vi "Main v1.5.vi"() -> ()   [LabVIEW 2017]
doc: "v0.85:\n- Counts for rejects and total\n\nv0.5:\n\n- Added Reject to Manual Mode\n- Send reject pallet cluster during manual mode\n- Run continuous manual happens only when no error has occured"
uses:
  Controls/Main Tabs v0.1.ctl
  Controls/Auto.ctl
  RT/Controls/Auto Delays.ctl
  RT/Controls/Auto Times.ctl
  support/Controls/General Para.ctl
  Controls/UI Data.ctl
  support/Controls/Auto Stats.ctl
  Controls/Logging FGV.ctl
  support/Message Queue/Enqueue Message (Single).vi
  GV/Maintenance GV.vi
  <vilib>/Utility/error.llb/Error Cluster From Error Code.vi
  <vilib>/ErrorRing/Error Ring.xnode
  support/Message Queue/Message Queue.lvlib
  support/User Event - Stop/User Event - Stop.lvlib
panel:
  out "path":path
  in  "General Para 2":T1={"Max. Cons."=5.0, "Offset 1"=0.0, "Offset 2"=0.0, "Offset 3"=0.0, "Offset 4"=-0.6, "OutputPause"=500.0, "RejectPause"=500.0} caption="General Para" {"Offset 4" format="%.2f"; "Offset 3" format="%.2f"; "Offset 2" format="%.2f"; "Offset 1" format="%.2f"}
  in  "Auto Para 2":T2={"Agitator Delays"=[250, 600], "TF Delays"=[400, 800, 2, 8000], "Insertion Delays"=[100, 400], "Cutting Delays"=[200, 300, 50], "PF Delays"=[300, 8000], "Measur. Delays"=[200.0, 188.9, 1.0], "Reject Delays"=[500], "BF Delays"=[1000, 1000]}
  out "Shutdown?":bool
  out "Boolean 8":bool
  out "Boolean 7":bool
  out "Boolean 6":bool
  out "Boolean 5":bool
  out "Boolean 4":bool
  out "Boolean 3":bool
  out "Boolean 2":bool
  out "Boolean":bool
  in  "Reject Pallets":T3
  out "Date-Time":string caption="Dip-Tube Assembly Automation (HMI) v1.5"
  out "Main Tab":T4
  in  "All IOs":bool
  in  "Autocycle":T5
  in  "Manual":bool
  in  "Parameters":bool
  in  "Maintenance":bool
  in  "General Para":T1={"Max. Cons."=5.0, "Offset 1"=0.0, "Offset 2"=0.0, "Offset 3"=0.0, "Offset 4"=0.0, "OutputPause"=0.0, "RejectPause"=0.0} {"Offset 4" format="%.2f"; "Offset 3" format="%.2f"; "Offset 2" format="%.2f"; "Offset 1" format="%.2f"}
  in  "BF Para":cluster{"Delay 1":u32, "Delay 2":u32}={"Delay 1"=1000, "Delay 2"=1000}
  in  "Reject Para":cluster{"Delay":u32}={"Delay"=400}
  in  "Meas. Para":T6={"Delay"=500.0, "Mean Length"=188.9, "Tolerance"=1.0}
  in  "PF Para":cluster{"Delay":u32, "Timeout":u32}={"Delay"=1000, "Timeout"=1000}
  in  "Tube Feeder Para":T7={"Delay"=400, "Delay 2"=250, "Max Attempts"=250, "Timeout"=8000}
  in  "Cutting Para":T8={"Delay"=400, "Delay 2"=250, "Delay 3"=250}
  in  "Agitator Para":cluster{"Delay":u32, "Timeout":u32}={"Delay"=400, "Timeout"=250}
  in  "Insertion Para":cluster{"Delay 1":u32, "Delay 2":u32}={"Delay 1"=1000, "Delay 2"=1000}
  in  "Save Para":bool
  in  "Home Para":bool
  out "OEE":dbl format="%#.1f"
  out "QUA":dbl=100.0 min=0.0 max=100.0 step=0.1
  in  "Ideal Time":dbl=2.0 min=0.0 max=100.0 step=0.1
  in  "AVL":dbl=100.0 min=0.0 max=100.0 step=0.1
  out "Rejects 2":u32 caption="Rejects"
  in  "Reset MCount":bool
  in  "Enable BF?":bool
  in  "Enable Agitate?":bool
  in  "Enable Reject?":bool
  in  "Toggle Motor":bool
  in  "Continuous?":bool
  in  "Enable Measure?":bool
  in  "Enable Index?":bool
  in  "Enable PF?":bool
  in  "Manual Para":T2={"Agitator Delays"=[400, 250], "TF Delays"=[700, 800, 2], "Insertion Delays"=[100, 500], "Cutting Delays"=[300, 300, 100], "PF Delays"=[250, 30000], "Measur. Delays"=[500.0, 188.9, 1.0], "Reject Delays"=[500], "BF Delays"=[1000, 1000]}
  in  "Enable Cutting?":bool
  in  "Enable Insertion?":bool
  in  "Run Manual":bool
  in  "Enable TF?":bool
  in  "Home Manual":bool
  out "Status 2":T10
  out "Measurements":T11 {"Height 1" format="%#.2f"; "Height 2" format="%#.2f"; "Height 3" format="%#.2f"; "Height 4" format="%#.2f"}
  out "Output Count":u32 caption="Output\nCount"
  out "PRF":dbl=100.0 min=0.0 max=100.0 step=0.1
  in  "End Cycle":bool
  out "Statuses":string[][](table)
  in  "All IO":bool
  in  "Stats":bool
  in  "Home AC":bool
  out "Status":string
  out "Good":u32 format="%06.0f"
  out "Cycle Time":dbl format="%0.2f"
  out "Rejects":u32 format="%06.0f"
  in  "View Log":bool
  out "Total Count 2":u32 caption="Total Count"
  out "Avg. Time":dbl caption="Avg. Cycle Time (s)" format="%#.3f"
  out "Output Chart":cluster{"Good Parts":u32, "Reject Parts":u32}(graph)
  out "Reject Count":u32
  out "Good Count":u32
  out "Total Time":dbl caption="Effective Cycle Time (s)" format="%#.3f"
  out "Time Chart":T12(graph)
  out "OEE Chart":T13(graph)
  out "Timestamp":string caption="Date & Timestamp"
  out "Latest Measure.":T14 caption="Latest Measurements" {"Length 1 (mm)" format="%#.2f"}
  out "Auto Times":T9
  in  "Back Stats":bool
  out "OEE 2":T13 caption="Latest Measurements" {"AVL" format="%#.1f"; "PRF" format="%#.1f"; "QUA" format="%#.1f"; "OEE" format="%#.1f"}
  out "Measurement Chart":T15(graph)
  in  "Home IOs":bool
  in  "Back IO":bool
  out "IAS 4":dbl format="%#.3f"
  out "IAS 3":dbl format="%#.3f"
  out "IAS 2":dbl format="%#.3f"
  out "IAS 1":dbl format="%#.3f"
  out "DI 1":T16
  out "DI 2":T17
  out "DO 1":T18
  in  "Exit":bool
  in  "Shutdown":bool
  # "HARMONY VISION DIP-TUBE ASSEMBLY AUTOMATION"
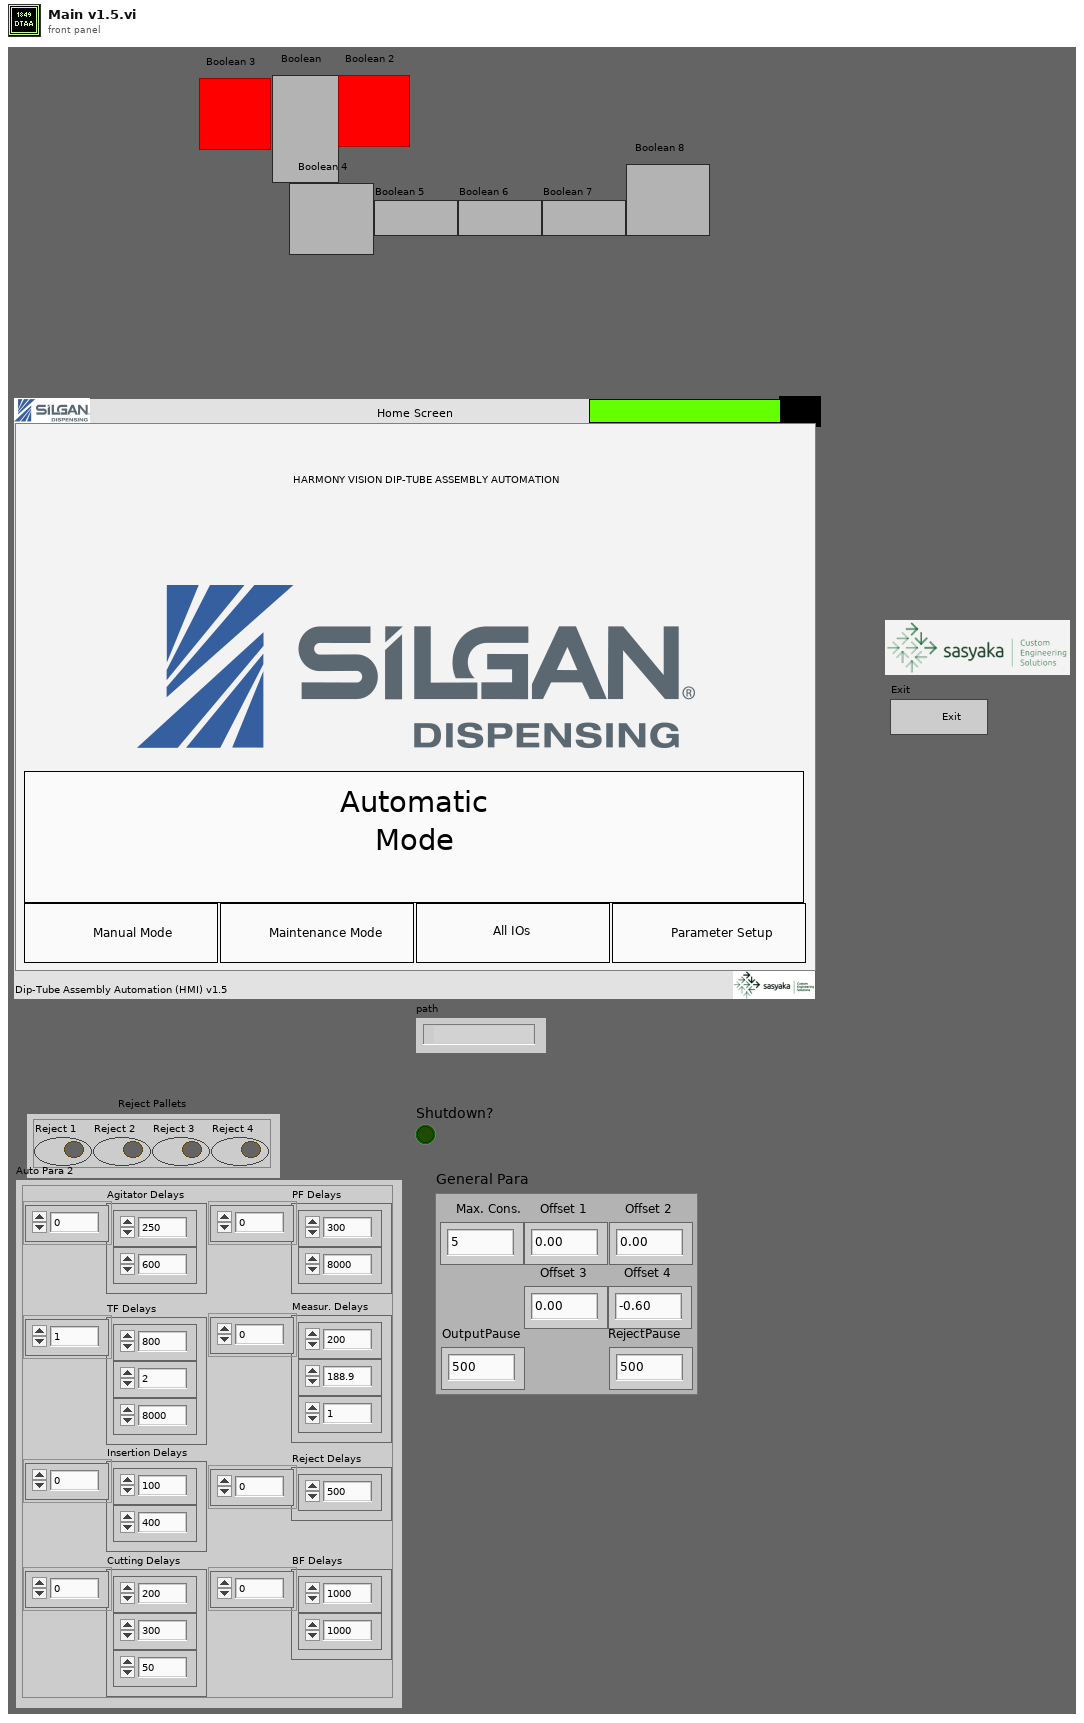
[diagram p1: front panel]
types:
  T1 = typedef "General Para.ctl" = cluster{"Max. Cons.":dbl, "Offset 1":dbl, "Offset 2":dbl, "Offset 3":dbl, "Offset 4":dbl, "OutputPause":dbl, "RejectPause":dbl}
  T2 = typedef "Auto Delays.ctl" = cluster{"Agitator Delays":u32[], "TF Delays":u32[], "Insertion Delays":u32[], "Cutting Delays":u32[], "PF Delays":u32[], "Measur. Delays":dbl[], "Reject Delays":u32[], "BF Delays":u32[]}
  T3 = cluster{"Reject 1":bool, "Reject 2":bool, "Reject 3":bool, "Reject 4":bool}
  T4 = typedef "Main Tabs v0.1.ctl" = enum32{"Home Screen", "Parameter Setup", "Manual Mode", "Autocycle", "Autocycle Statistics", "Autocycle IOs"}
  T5 = typedef "Auto.ctl" = bool
  T6 = cluster{"Delay":dbl, "Mean Length":dbl, "Tolerance":dbl}
  T7 = cluster{"Delay":u32, "Delay 2":u32, "Max Attempts":u32, "Timeout":u32}
  T8 = cluster{"Delay":u32, "Delay 2":u32, "Delay 3":u32}
  T9 = typedef "Auto Times.ctl" = cluster{"Index Time":u32, "TF Time":u32, "Insertion Time":u32, "Cutting Time":u32, "PF Time":u32, "Meas. Time":u32, "Reject Time":u32}
  T10 = cluster{"Auto Times":T9, "error out":errorcluster}
  T11 = cluster{"Height 1":dbl, "Height 2":dbl, "Height 3":dbl, "Height 4":dbl}
  T12 = cluster{"Index":dbl, "TF":dbl, "Insert":dbl, "Cutting":dbl, "PF":dbl, "Measure.":dbl, "Reject":dbl}
  T13 = cluster{"AVL":dbl, "PRF":dbl, "QUA":dbl, "OEE":dbl}
  T14 = cluster{"Length 1 (mm)":dbl, "Pallet 2 (mm)":dbl, "Pallet 3 (mm)":dbl, "Pallet 4 (mm)":dbl}
  T15 = cluster{"1":dbl, "2":dbl, "3":dbl, "4":dbl, "4":dbl, "4":dbl}
  T16 = cluster{"Machine_ON":bool, "E_stop ":bool, "SW_Pressure":bool, "SW_Start ":bool, "SW_Reset":bool, "SW_Stop":bool, "SW_Door":bool, "RS_Index_Rotary_CW":bool, "RS_Index_Rotary_CCW":bool, "RS_Index_Stopper _Rear":bool, "RS_Index_Output_Separator_Rear":bool, "PES_Index_Pallet_Sensor":bool, "PES_Index_Output_Part Sensor":bool, "ICS_BF_Low_Level_1":bool, "ICS_BF_Low_Level_2":bool, "ICS_BF_Pump_CNVR_Full_1":bool, "ICS_BF_Pump_CNVR_Full_2":bool, "ICS_BF_Pump_CNVR_Full_3":bool, "ICS_BF_Pump_CNVR_Full_4":bool, "PES_PC_Pump Presence_1":bool, "PES_PC_Pump Presence_2":bool, "PES_PC_Pump Presence_3":bool, "PES_PC_Pump Presence_4":bool, "RS_PC_Gating_Front":bool, "PES_Pump_Interference":bool, "PES_TF_Low_Level":bool, "PES_Tube Presence_1":bool, "PES_Tube Presence_2":bool, "PES_Tube Presence_3":bool, "PES_Tube Presence_4":bool, "DI1.30":bool, "DI1.31":bool}
  T17 = cluster{"RS_Agitatator_1_Rear ":bool, "RS_Agitatator_2_Rear ":bool, "RS_TF_Gating CYL_Rear":bool, "RS_Insertion_1_Rear":bool, "RS_Insertion_1_Front":bool, "RS_Insertion _2_Rear":bool, "RS_Insertion _2_Front":bool, "RS_Insertion _3_Rear":bool, "RS_Insertion _3_Front":bool, "RS_Insertion _4_Rear":bool, "RS_Insertion _4_Front":bool, "RS_Insertion_Clamp_Rear":bool, "RS_Cutting_Rear":bool, "RS_Cutting_Clamp _Rear":bool, "RS_Measurement_1_Rear":bool, "RS_Measurement_2_Rear":bool, "RS_Measurement_3_Rear":bool, "RS_Measurement_4_Rear":bool, "DI2.18":bool, "RS_Rejection_1_Rear":bool, "RS_Rejection_2_Rear":bool, "RS_Rejection_3_Rear":bool, "RS_Rejection_4_Rear":bool, "DI2.23":bool, "DI2.24":bool, "DI2.25":bool, "DI2.26":bool, "DI2.27":bool, "DI2.28":bool, "DI2.29":bool, "DI2.30":bool, "DI2.31":bool}
  T18 = cluster{"TL_Red":bool, "TL_Orange":bool, "TL_Green":bool, "TL_Buzzer":bool, "SOL_Index_Rotary_CW":bool, "SOL_Index_Rotary_CCW":bool, "SOL_Index_Stopper_Rear":bool, "SOL_OutputSeparator_Rear":bool, "Bowl  Feeder_ ON 1":bool, "Pump_CNVR_Motor _ON":bool, "SOL_PC_Gating_CYL_Rear":bool, "SOL_Tube_Feed_Agitatator":bool, "SOL_Tube_Feed_Gating_CYL":bool, "SOL_Insertion _CYL":bool, "SOL_Insertion_Clamp_CYL":bool, "SOL_Cutting_CYL":bool, "SOL_Cutting_Clamp_CYL":bool, "SOL_Insertion_Air_Nozzle":bool, "SOL_Measurement_CYL":bool, "DO1.19":bool, "SOL_Rejection CYL_1":bool, "SOL_Rejection CYL_2":bool, "SOL_Rejection CYL_3":bool, "SOL_Rejection CYL_4":bool, "Bowl  Feeder_ ON 2":bool, "SOL_BF_BlowerON":bool, "SOL_BF1_Track1":bool, "SOL_BF1_Track2":bool, "SOL_BF2_Track1":bool, "SOL_BF2_Track2":bool, "DO1.30":bool, "DO1.31":bool}
  T19 = typedef "UI Data.ctl" = cluster{"Main Tab":refnum<vi>}
  T20 = typedef "Message Queue.lvlib/All Message Queues.ctl" = cluster{"UI":refnum<queue>}
  T21 = enum8{"Enabled", "Disabled", "Disabled and Grayed Out"}
  T22 = cluster{"Array":string[][], "Machine Status":string}
  T23 = typedef "Logging FGV.ctl" = enum16{"Start Shift", "Log Index", "Read Shift", "Close Shift"}
  T24 = typedef "Auto Stats.ctl" = cluster{"Time-Stamp":timestamp, "Auto Times":T9, "Measurements":cluster{"1":dbl, "2":dbl, "3":dbl, "4":dbl}, "Outputs":cluster{"Good Parts":u32, "Reject Parts":u32}, "Cycle Time":dbl, "Remarks":string}
  T25 = cluster{"Auto Times":T9, "Results":cluster{"Measurements":cluster{"1":dbl, "2":dbl, "3":dbl, "4":dbl}, "Reject Pallets":cluster{"Reject 1":bool, "Reject 2":bool, "Reject 3":bool, "Reject 4":bool}}, "OutputCount":u32, "error out":errorcluster}
  T26 = enum8{"Information", "Error", "Successful", "Tips"}
  T27 = cluster{"Agitator Delays[0]":u32, "Agitator Delays[1]":u32}
  T28 = cluster{"TF Delays[0]":u32, "TF Delays[1]":u32, "TF Delays[2]":u32, "TF Delays[3]":u32}
  T29 = cluster{"Insertion Delays[0]":u32, "Insertion Delays[1]":u32}
  T30 = cluster{"Cutting Delays[0]":u32, "Cutting Delays[1]":u32, "Cutting Delays[2]":u32}
  T31 = cluster{"Measur. Delays[0]":dbl, "Measur. Delays[1]":dbl, "Measur. Delays[2]":dbl}
  T32 = typedef "All Inputs.ctl" = cluster{"DI 1":cluster{"Machine_ON":bool, "E_stop ":bool, "SW_Pressure":bool, "SW_Start ":bool, "SW_Reset":bool, "SW_Stop":bool, "SW_Door":bool, "RS_Index_Rotary_CW":bool, "RS_Index_Rotary_CCW":bool, "RS_Index_Stopper _Rear":bool, "RS_Cutting_DNClamp _Rear":bool, "PES_Index_Pallet_Sensor":bool, "PES_Index_Output_Part Sensor":bool, "ICS_BF_Low_Level_1":bool, "ICS_BF_Low_Level_2":bool, "ICS_BF_Pump_CNVR_Full_1":bool, "ICS_BF_Pump_CNVR_Full_2":bool, "ICS_BF_Pump_CNVR_Full_3":bool, "ICS_BF_Pump_CNVR_Full_4":bool, "PES_PC_Pump Presence_1":bool, "PES_PC_Pump Presence_2":bool, "PES_PC_Pump Presence_3":bool, "PES_PC_Pump Presence_4":bool, "RS_PC_Gating_Front":bool, "PES_Pump_Interference":bool, "PES_TF_Low_Level":bool, "PES_Tube Presence_1":bool, "PES_Tube Presence_2":bool, "PES_Tube Presence_3":bool, "PES_Tube Presence_4":bool, "DI1.30":bool, "DI1.31":bool}, "DI 2":cluster{"RS_Agitatator_1_Rear ":bool, "RS_Agitatator_2_Rear ":bool, "RS_TF_Gating CYL_Rear":bool, "RS_Insertion_1_Rear":bool, "RS_Insertion_1_Front":bool, "RS_Insertion _2_Rear":bool, "RS_Insertion _2_Front":bool, "RS_Insertion _3_Rear":bool, "RS_Insertion _3_Front":bool, "RS_Insertion _4_Rear":bool, "RS_Insertion _4_Front":bool, "RS_Insertion_Clamp_Rear":bool, "RS_Cutting_Rear":bool, "RS_Cutting_UPClamp _Rear":bool, "RS_Measurement_1_Rear":bool, "RS_Measurement_2_Rear":bool, "RS_Measurement_3_Rear":bool, "RS_Measurement_4_Rear":bool, "RS_Measure_Clamp_Rear":bool, "RS_Rejection_1_Rear":bool, "RS_Rejection_2_Rear":bool, "RS_Rejection_3_Rear":bool, "RS_Rejection_4_Rear":bool, "DI2.23":bool, "DI2.24":bool, "DI2.25":bool, "DI2.26":bool, "DI2.27":bool, "DI2.28":bool, "DI2.29":bool, "DI2.30":bool, "DI2.31":bool}, "IAS 1":dbl, "IAS 2":dbl, "IAS 3":dbl, "IAS 4":dbl, "DO 1":cluster{"TL_Red":bool, "TL_Orange":bool, "TL_Green":bool, "TL_Buzzer":bool, "SOL_Index_Rotary_CW":bool, "SOL_Index_CNVR_Rotary_CCW":bool, "SOL_Index_CNVR_Stopper_Rear":bool, "SOL_Index_CNVR_Output _Separator _Rear":bool, "Bowl  Feeder_ ON 1":bool, "Pump_CNVR_Motor _ON":bool, "SOL_PC_Gating_CYL_Rear":bool, "SOL_Tube_Feed_Agitatator":bool, "SOL_Tube_Feed_Gating_CYL":bool, "SOL_Insertion _CYL":bool, "SOL_Insertion_Clamp_CYL":bool, "SOL_Cutting_CYL":bool, "SOL_Cutting_Clamp_CYL":bool, "SOL_Insertion_Air_Nozzle":bool, "SOL_Measurement_CYL":bool, "DO1.19":bool, "SOL_Rejection CYL_1":bool, "SOL_Rejection CYL_2":bool, "SOL_Rejection CYL_3":bool, "SOL_Rejection CYL_4":bool, "Bowl  Feeder_ ON 2":bool, "SOL_BF_BlowerON":bool, "SOL_BF1_Track1":bool, "SOL_BF1_Track2":bool, "SOL_BF2_Track1":bool, "SOL_BF2_Track2":bool, "DO1.30":bool, "DO1.31":bool}}
  T33 = cluster{"Machine_ON":bool, "E_stop ":bool, "SW_Pressure":bool, "SW_Start ":bool, "SW_Reset":bool, "SW_Stop":bool, "SW_Door":bool, "RS_Index_Rotary_CW":bool, "RS_Index_Rotary_CCW":bool, "RS_Index_Stopper _Rear":bool, "RS_Cutting_DNClamp _Rear":bool, "PES_Index_Pallet_Sensor":bool, "PES_Index_Output_Part Sensor":bool, "ICS_BF_Low_Level_1":bool, "ICS_BF_Low_Level_2":bool, "ICS_BF_Pump_CNVR_Full_1":bool, "ICS_BF_Pump_CNVR_Full_2":bool, "ICS_BF_Pump_CNVR_Full_3":bool, "ICS_BF_Pump_CNVR_Full_4":bool, "PES_PC_Pump Presence_1":bool, "PES_PC_Pump Presence_2":bool, "PES_PC_Pump Presence_3":bool, "PES_PC_Pump Presence_4":bool, "RS_PC_Gating_Front":bool, "PES_Pump_Interference":bool, "PES_TF_Low_Level":bool, "PES_Tube Presence_1":bool, "PES_Tube Presence_2":bool, "PES_Tube Presence_3":bool, "PES_Tube Presence_4":bool, "DI1.30":bool, "DI1.31":bool}
  T34 = cluster{"RS_Agitatator_1_Rear ":bool, "RS_Agitatator_2_Rear ":bool, "RS_TF_Gating CYL_Rear":bool, "RS_Insertion_1_Rear":bool, "RS_Insertion_1_Front":bool, "RS_Insertion _2_Rear":bool, "RS_Insertion _2_Front":bool, "RS_Insertion _3_Rear":bool, "RS_Insertion _3_Front":bool, "RS_Insertion _4_Rear":bool, "RS_Insertion _4_Front":bool, "RS_Insertion_Clamp_Rear":bool, "RS_Cutting_Rear":bool, "RS_Cutting_UPClamp _Rear":bool, "RS_Measurement_1_Rear":bool, "RS_Measurement_2_Rear":bool, "RS_Measurement_3_Rear":bool, "RS_Measurement_4_Rear":bool, "RS_Measure_Clamp_Rear":bool, "RS_Rejection_1_Rear":bool, "RS_Rejection_2_Rear":bool, "RS_Rejection_3_Rear":bool, "RS_Rejection_4_Rear":bool, "DI2.23":bool, "DI2.24":bool, "DI2.25":bool, "DI2.26":bool, "DI2.27":bool, "DI2.28":bool, "DI2.29":bool, "DI2.30":bool, "DI2.31":bool}
  T35 = cluster{"TL_Red":bool, "TL_Orange":bool, "TL_Green":bool, "TL_Buzzer":bool, "SOL_Index_Rotary_CW":bool, "SOL_Index_CNVR_Rotary_CCW":bool, "SOL_Index_CNVR_Stopper_Rear":bool, "SOL_Index_CNVR_Output _Separator _Rear":bool, "Bowl  Feeder_ ON 1":bool, "Pump_CNVR_Motor _ON":bool, "SOL_PC_Gating_CYL_Rear":bool, "SOL_Tube_Feed_Agitatator":bool, "SOL_Tube_Feed_Gating_CYL":bool, "SOL_Insertion _CYL":bool, "SOL_Insertion_Clamp_CYL":bool, "SOL_Cutting_CYL":bool, "SOL_Cutting_Clamp_CYL":bool, "SOL_Insertion_Air_Nozzle":bool, "SOL_Measurement_CYL":bool, "DO1.19":bool, "SOL_Rejection CYL_1":bool, "SOL_Rejection CYL_2":bool, "SOL_Rejection CYL_3":bool, "SOL_Rejection CYL_4":bool, "Bowl  Feeder_ ON 2":bool, "SOL_BF_BlowerON":bool, "SOL_BF1_Track1":bool, "SOL_BF1_Track2":bool, "SOL_BF2_Track1":bool, "SOL_BF2_Track2":bool, "DO1.30":bool, "DO1.31":bool}
  T36 = cluster{"Manual Para":T2, "Reject Pallets":cluster{"Reject 1":bool, "Reject 2":bool, "Reject 3":bool, "Reject 4":bool}}
  T37 = cluster{"Measurements":cluster{"1":dbl, "2":dbl, "3":dbl, "4":dbl}, "Reject Pallets":cluster{"Reject 1":bool, "Reject 2":bool, "Reject 3":bool, "Reject 4":bool}}
  T38 = cluster{"Reject Pallets":cluster{"Reject 1":bool, "Reject 2":bool, "Reject 3":bool, "Reject 4":bool}, "Measurements":cluster{"1":dbl, "2":dbl, "3":dbl, "4":dbl}}
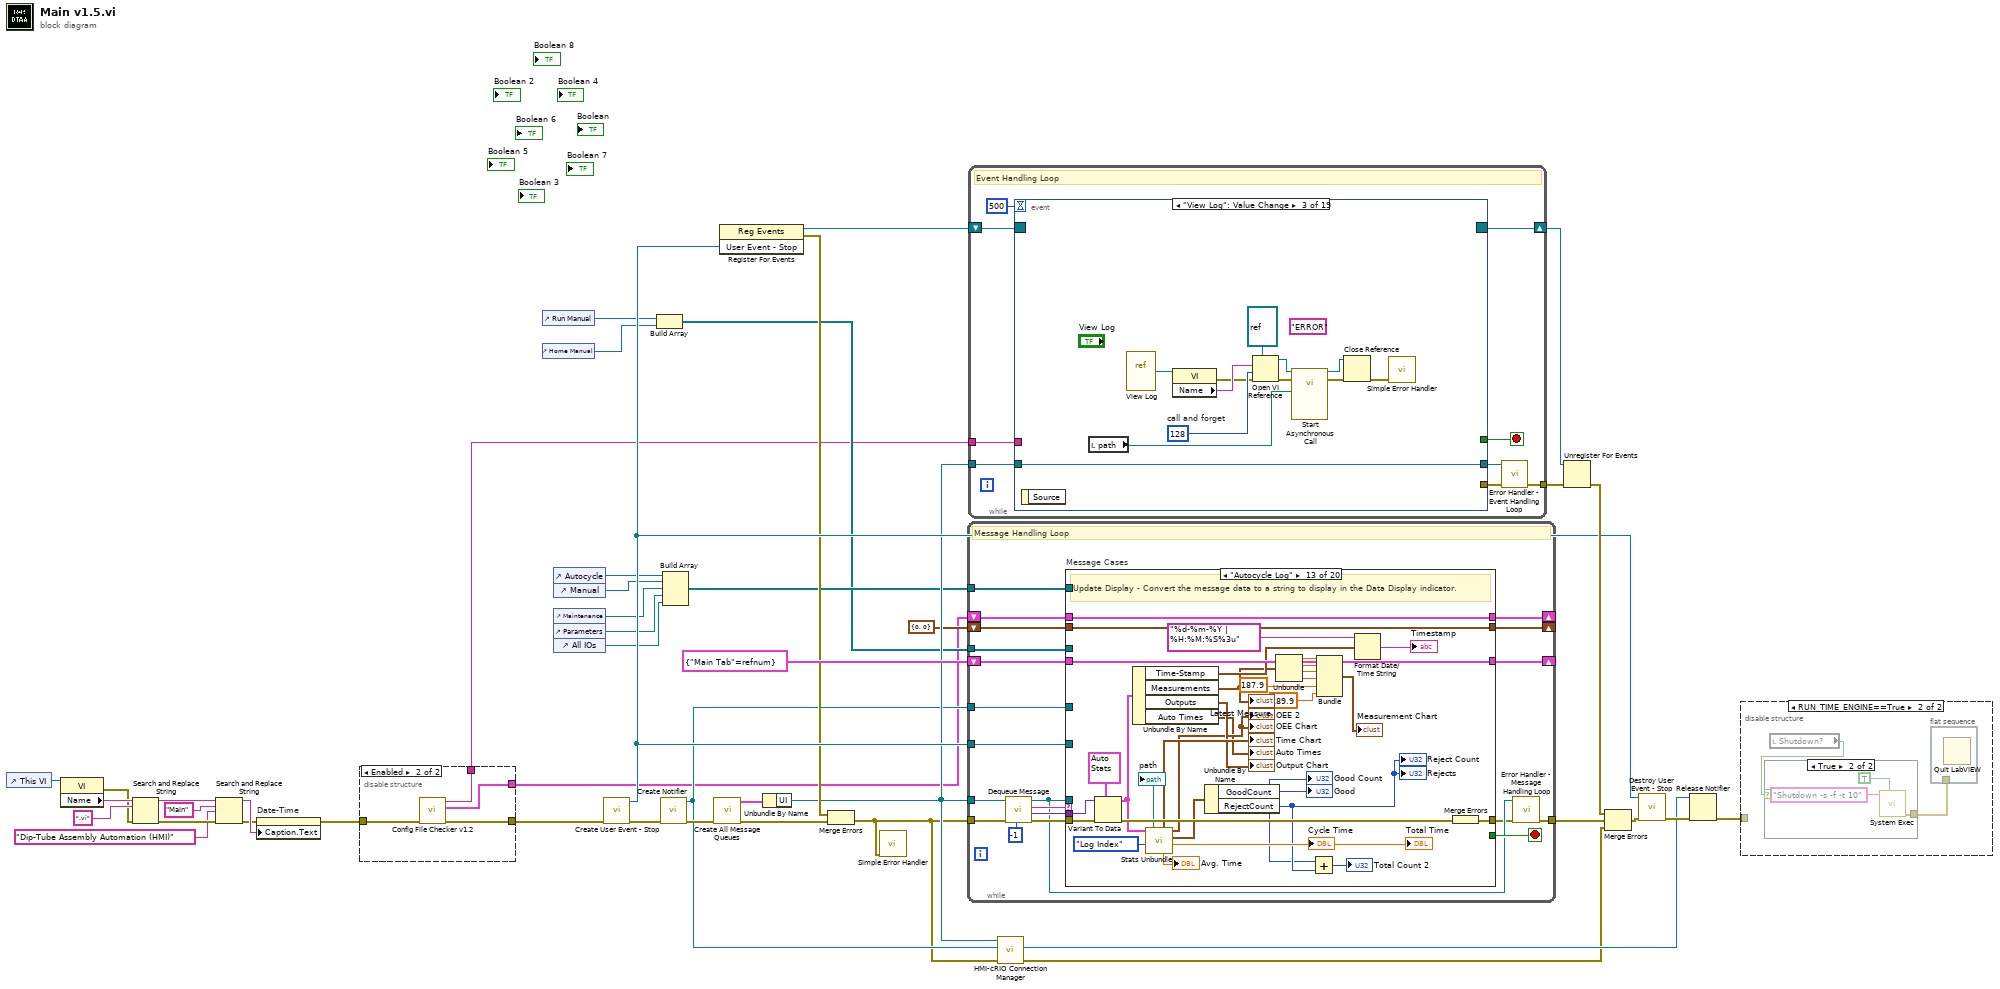
[diagram p0: block diagram]
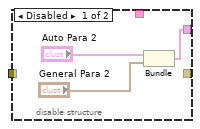
[diagram p2: hidden frame]
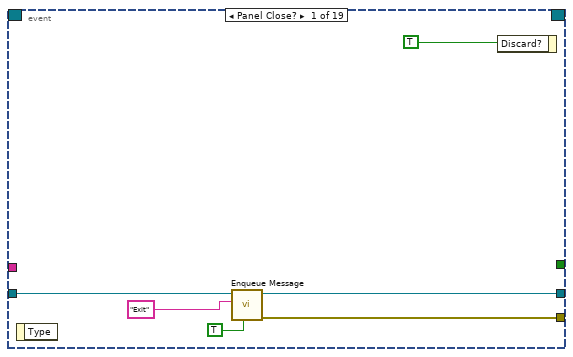
[diagram p3: hidden frame]
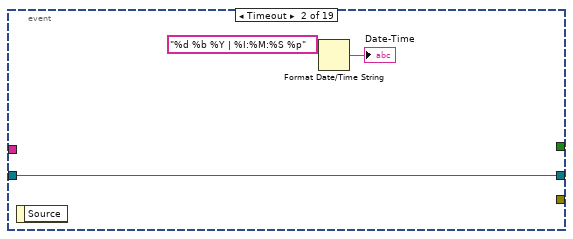
[diagram p4: hidden frame]
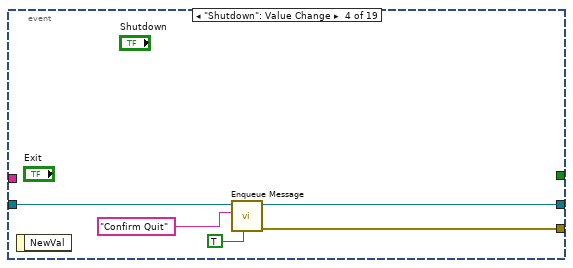
[diagram p5: hidden frame]
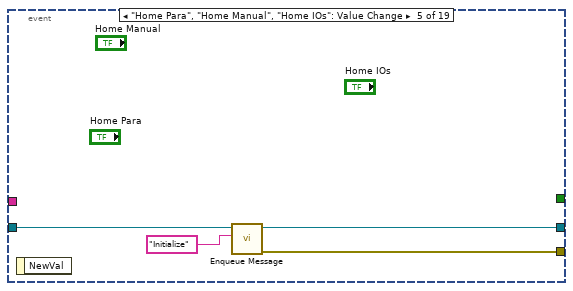
[diagram p6: hidden frame]
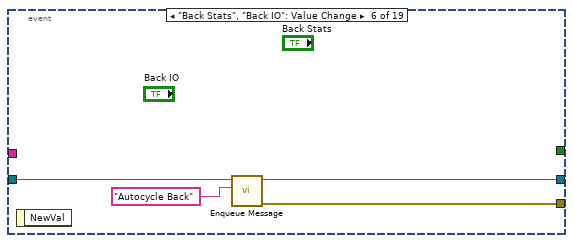
[diagram p7: hidden frame]
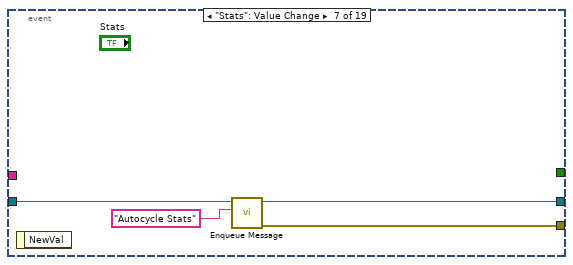
[diagram p8: hidden frame]
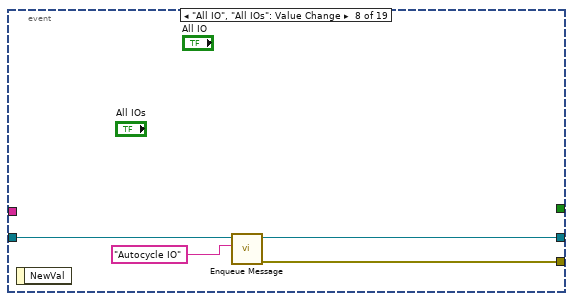
[diagram p9: hidden frame]
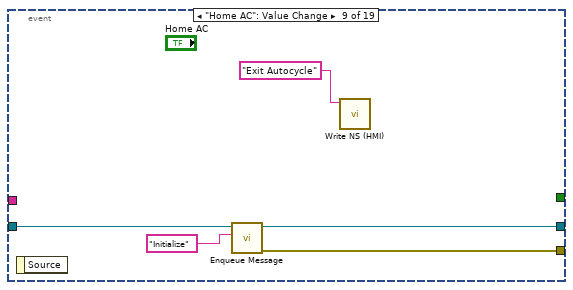
[diagram p10: hidden frame]
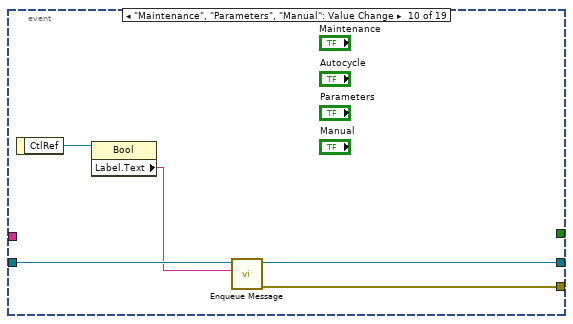
[diagram p11: hidden frame]
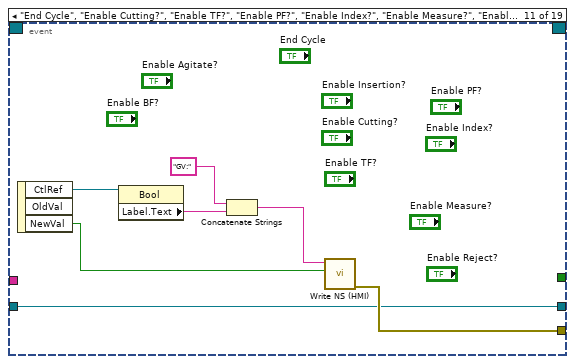
[diagram p12: hidden frame]
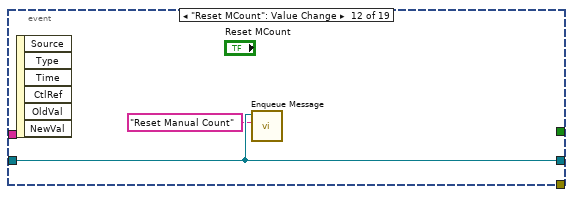
[diagram p13: hidden frame]
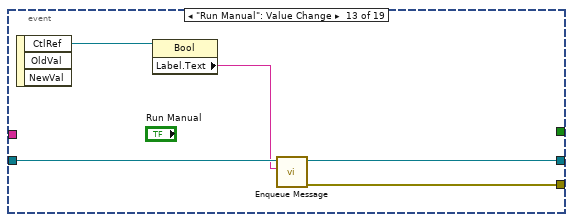
[diagram p14: hidden frame]
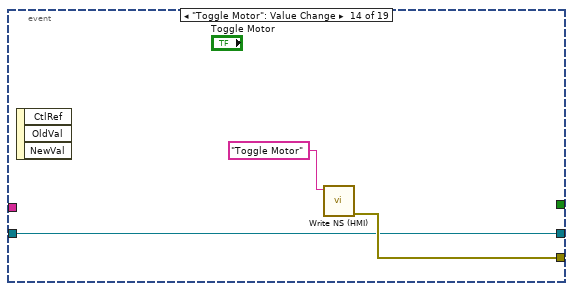
[diagram p15: hidden frame]
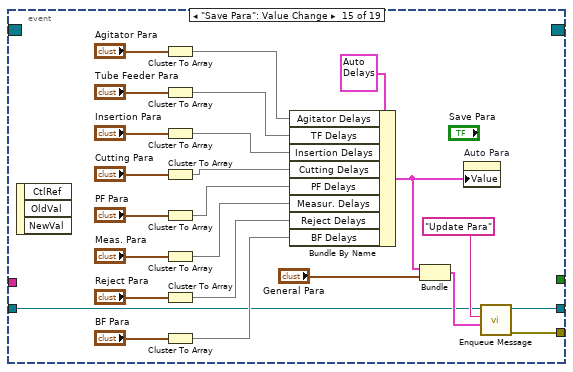
[diagram p16: hidden frame]
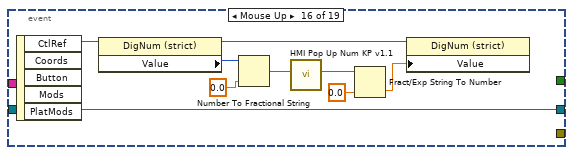
[diagram p17: hidden frame]
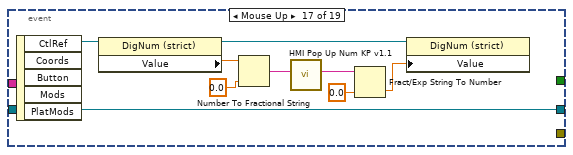
[diagram p18: hidden frame]
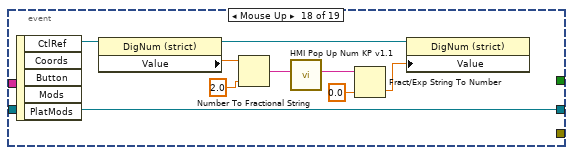
[diagram p19: hidden frame]
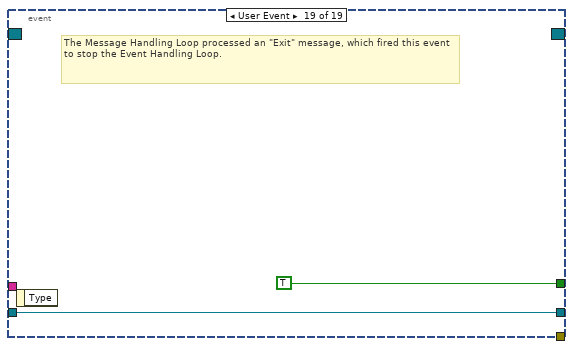
[diagram p20: hidden frame]
diagram:
  n1 = control-ref of="This VI"() -> (w15:refnum<vi>)
  n2 = property class="VI"(reference=w15) -> (error out=w14:errorcluster, "Name"=w21:string)  [unwired: 1 in, 1 out]
  n3 = Search and Replace String(input string=w21, search string=".vi", error in=w14) -> (result string=w19:string, error out=w18:errorcluster)  [unwired: 5 in, 2 out]
  n4 = Search and Replace String(input string=w19, search string="Main", replace string="Dip-Tube Assembly Automation (HMI)" ("replace string (\"\")"), error in=w18) -> (result string=w13:string, error out=w12:errorcluster)  [unwired: 4 in, 2 out]
  n5 = property on="Date-Time" class="Str"(error in=w12, "Caption.Text"=w13) -> (error out=w5:errorcluster)  [unwired: 1 in, 1 out]
  n6 = disable-structure shown="Enabled" {
    disable-tunnel: [w45 w51] -> w3
    disable-tunnel: w5 -> [_ w50]
    disable-tunnel: [_ w49] -> w4
    disable-tunnel: [_ w48] -> w2
    frame Disabled {
      n7 = Bundle("Auto Para 2"="Auto Para 2", "General Para 2"="General Para 2") -> (w45:cluster{"Auto Para 2":T2, "General Para 2":T1})  [unwired: 1 in]
    }
    frame Enabled {
      n8 = call "Config File Checker v1.2.vi"("Error In"=w50) -> ("error out"=w49:errorcluster, "All Para"=w51:cluster{"Auto Para":T2, "General Para 2":T1}, "password"=w48:string)  [unwired: 7 in, 1 out]
    }
  }
  n9 = control-ref of="Run Manual"() -> (w11:refnum<vi>)
  n10 = control-ref of="Home Manual"() -> (w10:refnum<vi>)
  n11 = control-ref of="Autocycle"() -> (w26:refnum<vi>)
  n12 = control-ref of="Manual"() -> (w25:refnum<vi>)
  n13 = control-ref of="Maintenance"() -> (w24:refnum<vi>)
  n14 = control-ref of="Parameters"() -> (w23:refnum<vi>)
  n15 = control-ref of="All IOs"() -> (w6:refnum<vi>)
  n16 = call "Create User Event - Stop.vi"("error in (no error)"=w4) -> ("error out"=w32:errorcluster, "User Event - Stop"=w35:refnum<user-event>)  [unwired: 9 in]
  n17 = Build Array(w11, w10) -> (w9:refnum<vi>[])
  n18 = call "Create Notifier.vi"("error in (no error)"=w32) -> ("error out"=w31:errorcluster, "notifier out"=w7:refnum<notifier>)  [unwired: 9 in]
  n19 = Build Array(w26, w25, w24, w23, w6) -> (w22:refnum<vi>[])
  n20 = call "Create All Message Queues.vi"("error in (no error)"=w31) -> ("error out"=w44:errorcluster, "Message Queues out"=w43:T20)  [unwired: 9 in]
  n21 = register-events(w35) -> (reference out=w36:refnum<event-registration>, error out=w34:errorcluster)  [unwired: 2 in]
  n22 = Unbundle By Name(w43) -> ("UI"=w33:refnum<queue>)
  n23 = Merge Errors(w34, w44) -> (w1:errorcluster)
  n24 = call <vilib>:"Simple Error Handler.vi"("error in (no error)"=w1) -> ()  [unwired: 4 in, 5 out]
  n25 = while {
    tunnel: w33 -> [w64]
    shift-right: [w71] -> _
    shift-left: T19 {"Main Tab"=refnum} ("Data Cluster") -> [w54]
    tunnel: w35 -> [w69]
    tunnel: w1 -> [w68]
    tunnel: [w62] -> w42
    tunnel: w7 -> [w59]
    tunnel: w22 -> [w58]
    tunnel: w9 -> [w57]
    shift-right: [w55] -> _
    shift-left: cluster{"OutputCount":u32, "RejectCount":u32} {"OutputCount"=0, "RejectCount"=0} -> [w56]
    shift-right: [w52] -> _
    shift-left: w3 -> [w53]
    stop <- w70 stop-if-true
    # "Message Handling Loop"
    n26 = call "Dequeue Message.vi"("timeout"=-1, "error in (no error)"=w68, "Message Queue"=w64) -> ("error out"=w67:errorcluster, "Message Data"=w65:variant, "Message"=w66:string, "dup Message Queue"=w63:refnum<queue>)  [unwired: 5 in]
    n27 = case "Message Cases" shown="\"Autocycle Log\"" w66 {
      selector: w66 -> [_ _ _ _ _ _ _ _ _ _ _ _ _ _ _ _ _ _ _ w387]
      tunnel: w63 -> [_ _ _ _ _ _ _ _ _ w192 w201 _ _ _ w306 _ _ w358 w384 _]
      tunnel: w67 -> [w80 w84 w99 w128 w139 w156 w164 w180 w186 w194 w209 w238 w270 w281 w314 w325 w349 w362 w377 _]
      tunnel: [w80 w83 w88 w128 w134 w156 w163 w180 w186 w193 w208 w239 w271 w283 w305 w325 w344 w360 w380 w388] -> w61
      tunnel: w54 -> [w79 w85 w101 w132 w141 w155 w160 w184 w190 w199 w206 w240 w272 w284 w315 w324 w348 w361 w383 w389]
      tunnel: [w78 w85 w101 w132 w141 w155 w160 w184 w190 w199 w206 w240 w272 w284 w315 w324 w348 w361 w383 w389] -> w71
      tunnel: [_ _ _ _ _ _ _ _ _ _ _ _ _ _ _ _ _ _ TRUE _] -> w70
      tunnel: w65 -> [_ _ w98 _ w138 _ _ _ _ _ _ w237 w269 _ w313 _ w347 _ w374 _]
      tunnel: w69 -> [_ _ _ _ _ _ _ _ _ _ _ _ _ _ _ _ _ _ w379 _]
      tunnel: w59 -> [_ _ _ _ _ _ _ _ _ _ _ _ _ _ _ _ _ _ w373 _]
      tunnel: w58 -> [_ _ w94 _ _ _ _ _ _ _ _ _ _ _ _ _ _ _ _ _]
      tunnel: w57 -> [_ _ _ _ _ _ _ _ _ _ _ _ _ w278 w311 _ _ _ _ _]
      tunnel: w56 -> [w75 w82 w90 w129 w140 w144 w165 w181 w187 w196 w210 w235 w267 w274 w304 _ w343 w357 w370 w386]
      tunnel: [w75 w82 w90 w129 w140 w144 w165 w181 w187 w196 w210 w235 w267 w274 w299 cluster{"OutputCount":u32, "RejectCount":u32} {"OutputCount"=0, "RejectCount"=0} w343 w357 w370 w386] -> w55
      tunnel: w53 -> [w72 w81 w87 w109 _ w143 w159 w179 w185 w191 w200 w224 w254 w273 w287 w321 w326 w350 w369 w385]
      tunnel: [w72 w81 w87 w109 w133 w143 w159 w179 w185 w191 w200 w224 w254 w273 w287 w321 w326 w350 w369 w385] -> w52
      frame "Initialize" {
        # "Initialize - All initialization work should take place in this message, since other loops can potentially enqueue messages that execute immediately after this one."
        n28 = control-ref of="Main Tab"() -> (w77:refnum<vi>)
        n29 = Bundle By Name(cluster=w79, "Main Tab"=w77) -> (w78:T19)
        n30 = property on="Home IOs" class="Bool"("Visible"=TRUE) -> ()  [unwired: 2 in, 2 out]
        n31 = property on="Back IO" class="Bool"("Visible"=FALSE) -> ()  [unwired: 2 in, 2 out]
        "Main Tab" <- Main_Tabs_v0.1."Home Screen" ("Main Tab")
      }
      frame "Maintenance" {
        # "Maintenance"
        n32 = call "Maintenance v0.3.vi"("Error In"=w84) -> ("Error out"=w83:errorcluster)  [unwired: 10 in]
      }
      frame "Connection" {
        n33 = Variant To Data(error in=w99, type=FALSE, Variant=w98) -> (data=w86:bool, error out=w89:errorcluster)
        n34 = Select(t=u32 6618880 ("Text.Text Colors:BG Color"), s=w86, f=u32 16762112 ("Text.Text Colors:BG Color")) -> (s? t:f=w95:u32)
        n35 = property on="Date-Time" class="Str"("Text.BGColor"=w95) -> ()  [unwired: 2 in, 2 out]
        n36 = Select(t=T21."Enabled" ("Disabled"), s=w86, f=T21."Disabled and Grayed Out") -> (s? t:f=w92:T21)
        n37 = for {
          tunnel: w94 -> [w108] mode=indexing
          tunnel: w92 -> [w107]
          n38 = property class="Bool"(reference=w108, "DisabledEnum"=w107) -> ()  [unwired: 1 in, 2 out]
        }
        n39 = case shown="True" w86 {
          tunnel: w89 -> [w102 w105]
          tunnel: [w102 w104] -> w88
          tunnel: w87 -> [_ w103]
          frame False {
          }
          frame True {
            n40 = call "Write NS (HMI).vi"("error in (no error)"=w105, "Message Data"=w103, "Message"="Save Para") -> ("error out"=w104:errorcluster)  [unwired: 8 in]
          }
        }
      }
      frame "Parameters" {
        # "Parameters"
        n41 = Unbundle(w109) -> ("Auto Para"=w111:T2, "General Para 2"=w110:T1)
        n42 = Unbundle By Name(w132) -> ("Main Tab"=w131:refnum<vi>)
        n43 = property on="General Para" class="Clust (strict)"("Value"=w110) -> ()  [unwired: 2 in, 2 out]
        n44 = Unbundle(w111) -> ("Agitator Delays"=w127:u32[], "TF Delays"=w126:u32[], "Insertion Delays"=w125:u32[], "Cutting Delays"=w124:u32[], "PF Delays"=w123:u32[], "Measur. Delays"=w122:dbl[], "Reject Delays"=w121:u32[], "BF Delays"=w120:u32[])
        n45 = property class="TabCtl"(reference=w131, "Value"=Main_Tabs_v0.1."Parameter Setup" ("Main Tab")) -> ()  [unwired: 1 in, 2 out]
        n46 = Array To Cluster(array=w127) -> (cluster=w119:T27)
        n47 = Array To Cluster(array=w126) -> (cluster=w118:T28)
        n48 = Array To Cluster(array=w125) -> (cluster=w117:T29)
        n49 = Array To Cluster(array=w124) -> (cluster=w116:T30)
        n50 = Array To Cluster(array=w123) -> (cluster=w115:cluster{"PF Delays[0]":u32, "PF Delays[1]":u32})
        n51 = Array To Cluster(array=w122) -> (cluster=w114:T31)
        n52 = Array To Cluster(array=w121) -> (cluster=w113:cluster{"Reject Delays[0]":u32})
        n53 = Array To Cluster(array=w120) -> (cluster=w112:cluster{"BF Delays[0]":u32, "BF Delays[1]":u32})
        n54 = property on="Agitator Para" class="Clust (strict)"("Value"=w119) -> ()  [unwired: 2 in, 2 out]
        n55 = property on="Tube Feeder Para" class="Clust (strict)"("Value"=w118) -> ()  [unwired: 2 in, 2 out]
        n56 = property on="Insertion Para" class="Clust (strict)"("Value"=w117) -> ()  [unwired: 2 in, 2 out]
        n57 = property on="Cutting Para" class="Clust (strict)"("Value"=w116) -> ()  [unwired: 2 in, 2 out]
        n58 = property on="PF Para" class="Clust (strict)"("Value"=w115) -> ()  [unwired: 2 in, 2 out]
        n59 = property on="Meas. Para" class="Clust (strict)"("Value"=w114) -> ()  [unwired: 2 in, 2 out]
        n60 = property on="Reject Para" class="Clust (strict)"("Value"=w113) -> ()  [unwired: 2 in, 2 out]
        n61 = property on="BF Para" class="Clust (strict)"("Value"=w112) -> ()  [unwired: 2 in, 2 out]
      }
      frame "Update Para" {
        # "Parameters"
        n62 = Variant To Data(error in=w139, type=cluster{"Auto Para":T2, "General Para":T1} {"Auto Para"={"Agitator Delays"=[], "TF Delays"=[], "Insertion Delays"=[], "Cutting Delays"=[], "PF Delays"=[], "Measur. Delays"=[], "Reject Delays"=[], "BF Delays"=[]}, "General Para"={"Max. Cons."=0.0, "Offset 1"=0.0, "Offset 2"=0.0, "Offset 3"=0.0, "Offset 4"=0.0, "OutputPause"=0.0, "RejectPause"=0.0}} ("cluster"), Variant=w138) -> (data=w133:cluster{"Auto Para":T2, "General Para":T1}, error out=w135:errorcluster)
        n63 = call "Write NS (HMI).vi"("error in (no error)"=w135, "Message Data"=w133, "Message"="Save Para") -> ("error out"=w134:errorcluster)  [unwired: 8 in]
      }
      frame "Manual" {
        # "Parameters"
        n64 = control-ref of="Enable Index?"() -> (w152:refnum<vi>)
        n65 = control-ref of="Enable PF?"() -> (w151:refnum<vi>)
        n66 = control-ref of="Enable Cutting?"() -> (w150:refnum<vi>)
        n67 = control-ref of="Enable Insertion?"() -> (w149:refnum<vi>)
        n68 = control-ref of="Enable TF?"() -> (w148:refnum<vi>)
        n69 = control-ref of="Enable Measure?"() -> (w146:refnum<vi>)
        n70 = Unbundle By Name(w143) -> ("Auto Para"=w142:T2)
        n71 = control-ref of="Enable Reject?"() -> (w145:refnum<vi>)
        n72 = Build Array(w152, w151, w150, w149, w148, w146, w145) -> (w147:refnum<vi>[])
        n73 = property on="Auto Para" class="Clust (strict)"("Value"=w142) -> ()  [unwired: 2 in, 2 out]
        n74 = for {
          tunnel: w147 -> [w158] mode=indexing
          n75 = property class="Bool (strict)"(reference=w158, "Val(Sgnl)"=FALSE ("Value (Signaling)")) -> ()  [unwired: 1 in, 2 out]
        }
        n76 = Unbundle By Name(w155) -> ("Main Tab"=w154:refnum<vi>)
        n77 = property class="TabCtl"(reference=w154, "Value"=Main_Tabs_v0.1."Manual Mode" ("Main Tab")) -> ()  [unwired: 1 in, 2 out]
      }
      frame "Autocycle" {
        # "Parameters"
        n78 = call "Select Model v0.1.vi"() -> ("Cancel out"=w161:bool, "Model out"=w162:string)  [unwired: 9 in, 1 out]
        n79 = case shown="False" w161 {
          tunnel: w164 -> [w169 w178]
          tunnel: [w176 w178] -> w163
          tunnel: w162 -> [w175 _]
          tunnel: w160 -> [w172 _]
          tunnel: w159 -> [w166 _]
          frame False {
            n80 = Unbundle By Name(w172) -> ("Main Tab"=w174:refnum<vi>)
            n81 = call "Write NS (HMI).vi"("error in (no error)"=w169, "Message Data"=w166, "Message"="Save Para") -> ("error out"=w168:errorcluster)  [unwired: 8 in]
            n82 = property class="TabCtl"(reference=w174, "Value"=Main_Tabs_v0.1."Autocycle" ("Main Tab")) -> ()  [unwired: 1 in, 2 out]
            n83 = call "Write NS (HMI).vi"("error in (no error)"=w168, "Message Data"=w175, "Message"="Autocycle") -> ("error out"=w176:errorcluster)  [unwired: 8 in]
            n84 = property on="Home IOs" class="Bool"("Visible"=FALSE) -> ()  [unwired: 2 in, 2 out]
            n85 = property on="Back IO" class="Bool"("Visible"=TRUE) -> ()  [unwired: 2 in, 2 out]
          }
          frame True {
          }
        }
      }
      frame "Autocycle Back" {
        # "Parameters"
        n86 = Unbundle By Name(w184) -> ("Main Tab"=w183:refnum<vi>)
        n87 = property class="TabCtl"(reference=w183, "Value"=Main_Tabs_v0.1."Autocycle" ("Main Tab")) -> ()  [unwired: 1 in, 2 out]
      }
      frame "Autocycle Stats" {
        # "Parameters"
        n88 = Unbundle By Name(w190) -> ("Main Tab"=w189:refnum<vi>)
        n89 = property class="TabCtl"(reference=w189, "Value"=Main_Tabs_v0.1."Autocycle Statistics" ("Main Tab")) -> ()  [unwired: 1 in, 2 out]
      }
      frame "Autocycle IO" {
        # "Parameters"
        n90 = Unbundle By Name(w199) -> ("Main Tab"=w198:refnum<vi>)
        n91 = property class="TabCtl"(reference=w198, "Value"=Main_Tabs_v0.1."Autocycle IOs" ("Main Tab")) -> ()  [unwired: 1 in, 2 out]
        n92 = call-poly "Enqueue Message.vi"("error in (no error)"=w194, "Message"="Update IO", "Message Queue"=w192) -> ("error out"=w193:errorcluster)  [unwired: 7 in, 1 out]
      }
      frame "Update IO" {
        n93 = Unbundle By Name(w206) -> ("Main Tab"=w207:refnum<vi>)
        n94 = Wait (ms)(milliseconds to wait=u32 200) -> ()  [unwired: 1 out]
        n95 = property class="TabCtl"(reference=w207) -> ("Value"=w205:variant)  [unwired: 1 in, 2 out]
        n96 = Variant To Data(type=Main_Tabs_v0.1."Autocycle IOs" ("Main Tab"), Variant=w205) -> (data=w202:T4)  [unwired: 1 in, 1 out]
        n97 = global read "Maintenance GV.vi" "All IO"() -> (w211:T32)
        n98 = case shown="\"Autocycle IOs\"" w202 {
          tunnel: w209 -> [w219 w222]
          tunnel: [w219 w221] -> w208
          tunnel: w201 -> [_ w220]
          frame Default {
          }
          frame "Autocycle IOs" {
            n99 = call-poly "Enqueue Message.vi"("error in (no error)"=w222, "Message"="Update IO", "Message Queue"=w220) -> ("error out"=w221:errorcluster)  [unwired: 7 in, 1 out]
          }
        }
        n100 = Unbundle(w211) -> ("DI 1"=→"DI 1":T33, "DI 2"=→"DI 2":T34, "IAS 1"=→"IAS 1":dbl, "IAS 2"=→"IAS 2":dbl, "IAS 3"=→"IAS 3":dbl, "IAS 4"=→"IAS 4":dbl, "DO 1"=→"DO 1":T35)
      }
      frame "Update UI" {
        # "Update Display - Convert the message data to a string to display in the Data Display indicator."
        n101 = Variant To Data(error in=w238, type=T22 {"Array"=[], "Machine Status"=""} ("Status Cluster"), Variant=w237) -> (data=w233:T22, error out=w236:errorcluster)
        n102 = Unbundle(w233) -> ("Array"=→"Statuses":string[][], "Machine Status"=w231:string)
        "Status" <- w231
        n103 = Search and Replace String(input string=w231, search string="Autocycle is Running") -> (number of replacements=w229:i32)  [unwired: 6 in, 3 out]
        n104 = Greater Than 0?(x=w229) -> (x > 0?=w227:bool)
        n105 = Select(t=T21."Disabled and Grayed Out" ("Disabled"), s=w227, f=T21."Enabled" ("Disabled")) -> (s? t:f=w226:T21)
        n106 = property on="Home AC" class="Bool"("DisabledEnum"=w226) -> ()  [unwired: 2 in, 2 out]
        n107 = Merge Errors(w236) -> (w239:errorcluster)
      }
      frame "Autocycle Log" {
        # "Update Display - Convert the message data to a string to display in the Data Display indicator."
        n108 = Variant To Data(error in=w270, type=T24 {"Time-Stamp"=timestamp(0 s since 1904-01-01), "Auto Times"={"Index Time"=0, "TF Time"=0, "Insertion Time"=0, "Cutting Time"=0, "PF Time"=0, "Meas. Time"=0, "Reject Time"=0}, "Measurements"={"1"=0.0, "2"=0.0, "3"=0.0, "4"=0.0}, "Outputs"={"Good Parts"=0, "Reject Parts"=0}, "Cycle Time"=0.0, "Remarks"=""} ("Auto Stats"), Variant=w269) -> (data=w265:T24, error out=w268:errorcluster)
        n109 = Unbundle By Name(w265) -> ("Time-Stamp"=w263:timestamp, "Measurements"=w253:cluster{"1":dbl, "2":dbl, "3":dbl, "4":dbl}, "Outputs"=→"Output Chart":cluster{"Good Parts":u32, "Reject Parts":u32}, "Auto Times"=→"Auto Times":T9)
        "Latest Measure." <- w253
        n110 = call "Stats Unbundle.vi"("State"=Logging_FGV."Log Index", "Auto Stats"=w265) -> ("Cycle Time"=→"Cycle Time" →"Total Time":dbl, "Counters"=w258:cluster{"GoodCount":u32, "RejectCount":u32}, "OEE Cluster"=→"OEE Chart" →"OEE 2":T13, "Avg. Cycle Time"=→"Avg. Time":dbl, "Total Times"=→"Time Chart":T12, "path"=→"path":path)  [unwired: 3 in, 1 out]
        n111 = Unbundle By Name(w258) -> ("GoodCount"=w242:u32, "RejectCount"=w243:u32)
        "Rejects" <- w243
        "Good" <- w242
        "Good Count" <- w242
        "Reject Count" <- w243
        n112 = Unbundle(w253) -> ("1"=w252:dbl, "2"=w251:dbl, "3"=w250:dbl, "4"=w249:dbl)
        n113 = Add(x=w242, y=w243) -> (x+y=→"Total Count 2":u32)
        n114 = Bundle("1"=w252, "2"=w251, "3"=w250, "4"=w249, "4"=187.9, "4"=189.9) -> (→"Measurement Chart":T15)  [unwired: 1 in]
        n115 = Format Date/Time String(time format string (%c)="%d-%m-%Y | %H:%M:%S%3u", seconds (now)=w263) -> (date/time string=→"Timestamp":string)  [unwired: 1 in]
        n116 = Merge Errors(w268) -> (w271:errorcluster)
      }
      frame "Run Manual" {
        # "Update Manual mode"
        n117 = Bundle("Manual Para"="Manual Para", "Reject Pallets"="Reject Pallets") -> (w275:T36)  [unwired: 1 in]
        n118 = for {
          tunnel: w278 -> [w286] mode=indexing
          tunnel: T21."Disabled and Grayed Out" ("Disabled") -> [w285]
          n119 = property class="Bool"(reference=w286, "DisabledEnum"=w285) -> ()  [unwired: 1 in, 2 out]
        }
        n120 = call "Write NS (HMI).vi"("error in (no error)"=w281, "Message Data"=w275, "Message"="Manual Run") -> ("error out"=w280:errorcluster)  [unwired: 8 in]
        n121 = Merge Errors(w280) -> (w283:errorcluster)
      }
      frame "Manual Status" {
        n122 = Variant To Data(error in=w314, type=T25 {"Auto Times"={"Index Time"=0, "TF Time"=0, "Insertion Time"=0, "Cutting Time"=0, "PF Time"=0, "Meas. Time"=0, "Reject Time"=0}, "Results"={"Measurements"={"1"=0.0, "2"=0.0, "3"=0.0, "4"=0.0}, "Reject Pallets"={"Reject 1"=FALSE, "Reject 2"=FALSE, "Reject 3"=FALSE, "Reject 4"=FALSE}}, "OutputCount"=0, "error out"={"status"=FALSE, "code"=0, "source"=""}} ("cluster"), Variant=w313) -> (data=w310:T25, error out=w305:errorcluster)
        n123 = Unbundle(w310) -> ("Auto Times"=w309:T9, "Results"=w301:T37, "OutputCount"=w300:u32, "error out"=w303:errorcluster)
        n124 = for {
          tunnel: w311 -> [w320] mode=indexing
          tunnel: T21."Enabled" ("Disabled") -> [w319]
          n125 = property class="Bool"(reference=w320, "DisabledEnum"=w319) -> ()  [unwired: 1 in, 2 out]
        }
        n126 = Unbundle(w301) -> ("Measurements"=w289:cluster{"1":dbl, "2":dbl, "3":dbl, "4":dbl}, "Reject Pallets"=w290:T3)
        "Measurements" <- w289
        n127 = Bundle("Auto Times"=w309, "error out"=w303) -> (→"Status 2":T10)  [unwired: 1 in]
        n128 = Bundle("Reject Pallets"=w290, "Measurements"=w289) -> (w288:T38)  [unwired: 1 in]
        n129 = call "Counts Update (manual).vi"("output cluster"=w288, "Desired Cycle Time (s)"="Ideal Time", "AVL"="AVL", "OutputCount"=w300, "Counts in"=w304) -> ("OEE"=w294:T13, "Counts out"=w299:cluster{"OutputCount":u32, "RejectCount":u32})  [unwired: 5 in]
        n130 = Unbundle(w294) -> ("PRF"=→"PRF":dbl, "QUA"=→"QUA":dbl, "OEE"=→"OEE":dbl)  [unwired: 1 out]
        n131 = Unbundle(w299) -> ("OutputCount"=→"Output Count":u32, "RejectCount"=→"Rejects 2":u32)
        n132 = case shown="True" "Continuous?" {
          tunnel: w306 -> [_ w318]
          tunnel: w303 -> [_ w317]
          frame False {
          }
          frame True {
            # "Run if continuous is TRUE & No Error"
            n133 = call-poly "Enqueue Message.vi"("error in (no error)"=w317, "Message"="Run Manual", "Message Queue"=w318) -> ()  [unwired: 7 in, 2 out]
          }
        }
      }
      frame "Reset Manual Count" {
        w322 = u32 0 ("Rejects")
        n134 = local write "Rejects 2"(w322) -> ()
        n135 = local write "Output Count"(w322) -> ()
      }
      frame "Error" {
        w330 = 128  # call and forget
        # "Run async so that this loop will continue to run"
        # "Error"
        n136 = Variant To Data(error in=w349, type=errorcluster {"status"=FALSE, "code"=0, "source"=""} ("error constant"), Variant=w347) -> (data=w342:errorcluster, error out=w345:errorcluster)
        n137 = Unbundle By Name(w342) -> ("source"=w341:string)
        n138 = vi-ref "NewDialog.vi"() -> (w337:refnum<vi>)
        n139 = property class="VI"(reference=w337) -> (error out=w339:errorcluster, "Name"=w338:string)  [unwired: 1 in, 1 out]
        n140 = Search and Replace String(input string=w341, search string="<err>") -> (result string=w329:string)  [unwired: 6 in, 3 out]
        n141 = Open VI Reference(type specifier VI Refnum (for type only)=refnum<vi> refnum, vi path=w338, options=w330, error in (no error)=w339) -> (vi reference=w332:refnum<vi>, error out=w333:errorcluster)  [unwired: 2 in]
        n142 = call-by-ref "Start Asynchronous Call"(reference=w332, error in=w333, "inIcon"=T26."Error", "inTitle"="ERROR", "inMessage"=w329) -> (reference out=w335:refnum<vi>, error out=w334:errorcluster)  [unwired: 6 in, 3 out]
        n143 = Close Reference(reference=w335, error in (no error)=w334) -> (error out=w336:errorcluster)
        n144 = call <vilib>:"Simple Error Handler.vi"("error in (no error)"=w336) -> ()  [unwired: 4 in, 5 out]
        n145 = Merge Errors(w345) -> (w344:errorcluster)
      }
      frame "Confirm Quit" {
        # "Confirm Quit - Message that can confirm whether or not the user wants to exit the application."
        n146 = call "NewDialog.vi"("inIcon"=T26."Information", "inTitle"="SHUTDOWN?", "inButton2Text"="Shutdown", "inButton1Text"="", "inMessage"="Are you sure you want to shutdown?") -> ("outButton2"=w351:bool)  [unwired: 4 in, 2 out]
        "Shutdown?" <- w351
        n147 = case shown="True" w351 {
          tunnel: w362 -> [w363 w368]
          tunnel: [w363 w367] -> w359
          tunnel: w358 -> [_ w366]
          frame False {
          }
          frame True {
            n148 = call-poly "Enqueue Message.vi"("Priority Message? (F)"=TRUE, "error in (no error)"=w368, "Message"="Exit", "Message Queue"=w366) -> ("error out"=w367:errorcluster)  [unwired: 6 in, 1 out]
          }
        }
        n149 = Merge Errors(w359) -> (w360:errorcluster)
      }
      frame "Exit" {
        # "Stop the VI"
        # "Release the message queue reference"
        # "Exit - Exit the application."
        n150 = Variant To Data(type=errorcluster {"status"=FALSE, "code"=0, "source"=""} ("error constant"), Variant=w374) -> (data=w375:errorcluster)  [unwired: 1 in, 1 out]
        n151 = call <vilib>:"Simple Error Handler.vi"("error in (no error)"=w375) -> ()  [unwired: 4 in, 5 out]
        n152 = Send Notification(notification=TRUE, notifier=w373) -> (error out=w371:errorcluster)  [unwired: 1 in, 1 out]
        n153 = call "Fire User Event - Stop.vi"("User Event - Stop"=w379) -> ("error out"=w378:errorcluster)  [unwired: 10 in]
        n154 = Release Queue(queue=w384, error in (no error)=w377) -> (error out=w381:errorcluster)  [unwired: 1 in, 2 out]
        n155 = Merge Errors(w371, w378, w381) -> (w380:errorcluster)
      }
      frame Default {
        # "'Default' case only runs if there is a message that isn't defined in any of the other cases.  Output a programming error."
        n156 = xnode "Error Ring"("parameter 0"=w387) -> ("error out"=w388:errorcluster)
      }
    }
    n157 = call "Error Handler - Message Handling Loop.vi"("error in (no error)"=w61, "Message Queue"=w63) -> ("dup error in"=w62:errorcluster)  [unwired: 8 in, 1 out]
  }
  n158 = while {
    tunnel: w33 -> [w405]
    shift-right: [w403] -> w39
    shift-left: w36 -> [w404]
    tunnel: [w399] -> w37
    tunnel: w2 -> [w397]
    stop <- w401 stop-if-true
    # "Event Handling Loop"
    n159 = event shown="[2] \"View Log\": Value Change" {
      selector: w404 -> [_ _ _ _ _ _ _ _ _ _ _ _ _ _ _ _ _ _ _]
      dyn-events: [_ _ _ _ _ _ _ _ _ _ _ _ _ _ _ _ _ _ _] -> w403
      timeout: 500 -> [_ _ _ _ _ _ _ _ _ _ _ _ _ _ _ _ _ _ _]
      tunnel: [_ _ _ _ _ _ _ _ _ _ _ _ _ _ _ _ _ _ TRUE ("Discard?")] -> w401
      tunnel: w405 -> [w410 w414 w426 w431 w435 w439 w443 w447 w452 w457 w462 w466 w471 w473 w476 w507 w516 w525 w527]
      tunnel: [w409 _ _ w430 w434 w438 w442 w446 w451 w456 w463 _ w469 w474 w479 _ _ _ _] -> w402
      tunnel: [w408 w414 w426 w429 w433 w437 w441 w445 w450 w455 w462 w466 w470 w473 w475 w507 w516 w525 w527] -> w400
      tunnel: w397 -> [_ _ _ _ _ _ _ _ _ _ _ _ _ _ _ _ _ _ _]
      event Panel Close? {
        n160 = event-data() -> ()  [unwired: 1 in, 1 out]
        n161 = call-poly "Enqueue Message.vi"("Priority Message? (F)"=TRUE, "Message"="Exit", "Message Queue"=w410) -> ("error out"=w409:errorcluster, "dup Message Queue"=w408:refnum<queue>)  [unwired: 7 in]
        n162 = event-data("Discard?"=TRUE) -> ()  [unwired: 1 in, 1 out]
      }
      event Timeout {
        n163 = event-data() -> ()  [unwired: 1 in, 1 out]
        n164 = Format Date/Time String(time format string (%c)="%d %b %Y | %I:%M:%S %p") -> (date/time string=→"Date-Time":string)  [unwired: 2 in]
      }
      event "View Log": Value Change {
        (unwired) "ERROR" ("inTitle")
        w425 = 128  # call and forget
        n165 = event-data() -> ()  [unwired: 1 in, 1 out]
        n166 = local read "path"() -> (w415:path)
        n167 = vi-ref "View Log.vi"() -> (w418:refnum<vi>)
        n168 = property class="VI"(reference=w418) -> (error out=w416:errorcluster, "Name"=w417:string)  [unwired: 1 in, 1 out]
        n169 = Open VI Reference(type specifier VI Refnum (for type only)=refnum<vi> refnum, vi path=w417, options=w425, error in (no error)=w416) -> (vi reference=w423:refnum<vi>, error out=w422:errorcluster)  [unwired: 2 in]
        n170 = call-by-ref "Start Asynchronous Call"(reference=w423, error in=w422, "file path"=w415) -> (reference out=w420:refnum<vi>, error out=w421:errorcluster)  [unwired: 10 in, 1 out]
        n171 = Close Reference(reference=w420, error in (no error)=w421) -> (error out=w419:errorcluster)
        n172 = call <vilib>:"Simple Error Handler.vi"("error in (no error)"=w419) -> ()  [unwired: 4 in, 5 out]
      }
      event "Shutdown": Value Change {
        n173 = event-data() -> ()  [unwired: 1 in, 1 out]
        n174 = call-poly "Enqueue Message.vi"("Priority Message? (F)"=TRUE, "Message"="Confirm Quit", "Message Queue"=w431) -> ("error out"=w430:errorcluster, "dup Message Queue"=w429:refnum<queue>)  [unwired: 7 in]
      }
      event "Home Para", "Home Manual", "Home IOs": Value Change {
        n175 = event-data() -> ()  [unwired: 1 in, 1 out]
        n176 = call-poly "Enqueue Message.vi"("Message"="Initialize", "Message Queue"=w435) -> ("error out"=w434:errorcluster, "dup Message Queue"=w433:refnum<queue>)  [unwired: 8 in]
      }
      event "Back Stats", "Back IO": Value Change {
        n177 = event-data() -> ()  [unwired: 1 in, 1 out]
        n178 = call-poly "Enqueue Message.vi"("Message"="Autocycle Back", "Message Queue"=w439) -> ("error out"=w438:errorcluster, "dup Message Queue"=w437:refnum<queue>)  [unwired: 8 in]
      }
      event "Stats": Value Change {
        n179 = event-data() -> ()  [unwired: 1 in, 1 out]
        n180 = call-poly "Enqueue Message.vi"("Message"="Autocycle Stats", "Message Queue"=w443) -> ("error out"=w442:errorcluster, "dup Message Queue"=w441:refnum<queue>)  [unwired: 8 in]
      }
      event "All IO", "All IOs": Value Change {
        n181 = event-data() -> ()  [unwired: 1 in, 1 out]
        n182 = call-poly "Enqueue Message.vi"("Message"="Autocycle IO", "Message Queue"=w447) -> ("error out"=w446:errorcluster, "dup Message Queue"=w445:refnum<queue>)  [unwired: 8 in]
      }
      event "Home AC": Value Change {
        n183 = event-data() -> ()  [unwired: 1 in, 1 out]
        n184 = call-poly "Enqueue Message.vi"("Message"="Initialize", "Message Queue"=w452) -> ("error out"=w451:errorcluster, "dup Message Queue"=w450:refnum<queue>)  [unwired: 8 in]
        n185 = call "Write NS (HMI).vi"("Message"="Exit Autocycle") -> ()  [unwired: 10 in, 1 out]
      }
      event "Maintenance", "Parameters", "Manual": Value Change {
        n186 = event-data() -> ("CtlRef"=w454:refnum<vi>)  [unwired: 1 in]
        n187 = property class="Bool"(reference=w454) -> ("Label.Text"=w453:string)  [unwired: 1 in, 2 out]
        n188 = call-poly "Enqueue Message.vi"("Message"=w453, "Message Queue"=w457) -> ("error out"=w456:errorcluster, "dup Message Queue"=w455:refnum<queue>)  [unwired: 8 in]
      }
      event "End Cycle", "Enable Cutting?", "Enable TF?", "Enable PF?", "Enable Index?", "Enable Measure?", "Enable Reject?", "Enable Agitate?", "Enable BF?", "Enable Insertion?": Value Change {
        n189 = event-data() -> ("CtlRef"=w464:refnum<vi>, "NewVal"=w458:bool)  [unwired: 1 in, 1 out]
        n190 = property class="Bool"(reference=w464) -> ("Label.Text"=w461:string)  [unwired: 1 in, 2 out]
        n191 = Concatenate Strings("GV:" ("string"), w461) -> (w459:string)
        n192 = call "Write NS (HMI).vi"("Message Data"=w458, "Message"=w459) -> ("error out"=w463:errorcluster)  [unwired: 9 in]
      }
      event "Reset MCount": Value Change {
        n193 = event-data() -> ()  [unwired: 1 in, 6 out]
        n194 = call-poly "Enqueue Message.vi"("Message"="Reset Manual Count", "Message Queue"=w466) -> ()  [unwired: 8 in, 2 out]
      }
      event "Run Manual": Value Change {
        n195 = event-data() -> ("CtlRef"=w468:refnum<vi>)  [unwired: 1 in, 2 out]
        n196 = property class="Bool"(reference=w468) -> ("Label.Text"=w467:string)  [unwired: 1 in, 2 out]
        n197 = call-poly "Enqueue Message.vi"("Message"=w467, "Message Queue"=w471) -> ("error out"=w469:errorcluster, "dup Message Queue"=w470:refnum<queue>)  [unwired: 8 in]
      }
      event "Toggle Motor": Value Change {
        n198 = event-data() -> ()  [unwired: 1 in, 3 out]
        n199 = call "Write NS (HMI).vi"("Message"="Toggle Motor") -> ("error out"=w474:errorcluster)  [unwired: 10 in]
      }
      event "Save Para": Value Change {
        n200 = event-data() -> ()  [unwired: 1 in, 3 out]
        n201 = Cluster To Array(cluster="Agitator Para") -> (array=w496:u32[])
        n202 = Cluster To Array(cluster="Tube Feeder Para") -> (array=w494:u32[])
        n203 = Cluster To Array(cluster="Insertion Para") -> (array=w492:u32[])
        n204 = Cluster To Array(cluster="Cutting Para") -> (array=w490:u32[])
        n205 = Cluster To Array(cluster="PF Para") -> (array=w488:u32[])
        n206 = Cluster To Array(cluster="Meas. Para") -> (array=w486:dbl[])
        n207 = Cluster To Array(cluster="Reject Para") -> (array=w484:u32[])
        n208 = Cluster To Array(cluster="BF Para") -> (array=w482:u32[])
        n209 = Bundle By Name(cluster=T2 {"Agitator Delays"=[1000], "TF Delays"=[1000], "Insertion Delays"=[1000], "Cutting Delays"=[1000], "PF Delays"=[1000], "Measur. Delays"=[1000.0], "Reject Delays"=[1000], "BF Delays"=[1000]} ("Auto Para"), "Agitator Delays"=w496, "TF Delays"=w494, "Insertion Delays"=w492, "Cutting Delays"=w490, "PF Delays"=w488, "Measur. Delays"=w486, "Reject Delays"=w484, "BF Delays"=w482) -> (w481:T2)
        n210 = Bundle("Auto Para"=w481, "General Para"="General Para") -> (w478:cluster{"Auto Para":T2, "General Para":T1})  [unwired: 1 in]
        n211 = property on="Auto Para" class="Clust (strict)"("Value"=w481) -> ()  [unwired: 2 in, 2 out]
        n212 = call-poly "Enqueue Message.vi"("Message Data"=w478, "Message"="Update Para", "Message Queue"=w476) -> ("error out"=w479:errorcluster, "dup Message Queue"=w475:refnum<queue>)  [unwired: 7 in]
      }
      event "Insertion Para.Delay 1", "Insertion Para.Delay 2", "Agitator Para.Delay", "Agitator Para.Timeout", "Cutting Para.Delay", "Cutting Para.Delay 2", "Cutting Para.Delay 3", "Tube Feeder Para.Delay", "Tube Feeder Para.Delay 2", "Tube Feeder Para.Max Attempts", "PF Para.Delay", "PF Para.Timeout", "Reject Para.Delay", "BF Para.Delay 1", "BF Para.Delay 2": Mouse Up {
        n213 = event-data() -> ("CtlRef"=w499:refnum<vi>)  [unwired: 1 in, 4 out]
        n214 = property class="DigNum (strict)"(reference=w499) -> (reference out=w502:refnum<vi>, "Value"=w503:u32)  [unwired: 1 in, 1 out]
        n215 = Number To Fractional String(number=w503, precision (6)=0.0 ("width (-)")) -> (F-format string=w501:string)  [unwired: 2 in]
        n216 = call "HMI Pop Up Num KP v1.1.vi"("String In"=w501) -> ("String Out"=w500:string)  [unwired: 9 in, 1 out]
        n217 = Fract/Exp String To Number(string=w500, default (0 dbl)=0.0 ("default (0 I32)")) -> (number=w505:dbl)  [unwired: 2 in, 1 out]
        n218 = property class="DigNum (strict)"(reference=w502, "Value"=w505) -> ()  [unwired: 1 in, 2 out]
      }
      event "Meas. Para.Delay": Mouse Up {
        n219 = event-data() -> ("CtlRef"=w508:refnum<vi>)  [unwired: 1 in, 4 out]
        n220 = property class="DigNum (strict)"(reference=w508) -> (reference out=w511:refnum<vi>, "Value"=w512:dbl)  [unwired: 1 in, 1 out]
        n221 = Number To Fractional String(number=w512, precision (6)=0.0 ("width (-)")) -> (F-format string=w510:string)  [unwired: 2 in]
        n222 = call "HMI Pop Up Num KP v1.1.vi"("String In"=w510) -> ("String Out"=w509:string)  [unwired: 9 in, 1 out]
        n223 = Fract/Exp String To Number(string=w509, default (0 dbl)=0.0 ("default (0 I32)")) -> (number=w514:dbl)  [unwired: 2 in, 1 out]
        n224 = property class="DigNum (strict)"(reference=w511, "Value"=w514) -> ()  [unwired: 1 in, 2 out]
      }
      event "Meas. Para.Mean Length", "Meas. Para.Tolerance": Mouse Up {
        n225 = event-data() -> ("CtlRef"=w517:refnum<vi>)  [unwired: 1 in, 4 out]
        n226 = property class="DigNum (strict)"(reference=w517) -> (reference out=w520:refnum<vi>, "Value"=w521:dbl)  [unwired: 1 in, 1 out]
        n227 = Number To Fractional String(number=w521, precision (6)=2.0 ("width (-)")) -> (F-format string=w519:string)  [unwired: 2 in]
        n228 = call "HMI Pop Up Num KP v1.1.vi"("String In"=w519) -> ("String Out"=w518:string)  [unwired: 9 in, 1 out]
        n229 = Fract/Exp String To Number(string=w518, default (0 dbl)=0.0 ("default (0 I32)")) -> (number=w523:dbl)  [unwired: 2 in, 1 out]
        n230 = property class="DigNum (strict)"(reference=w520, "Value"=w523) -> ()  [unwired: 1 in, 2 out]
      }
      event User Event {
        # "The Message Handling Loop processed an \"Exit\" message, which fired this event to stop the Event Handling Loop."
        n231 = event-data() -> ()  [unwired: 1 in, 1 out]
      }
    }
    n232 = call "Error Handler - Event Handling Loop.vi"("error in (no error)"=w402, "Message Queue"=w400) -> ("dup error in"=w399:errorcluster)  [unwired: 8 in, 1 out]
  }
  n233 = call "HMI-cRIO Connection Manager.vi"("error in"=w1, "notifier in"=w7, "Queue in"=w33) -> ("error out"=w27:errorcluster, "Notifier out"=w28:refnum<notifier>)  [unwired: 7 in]
  n234 = Unregister For Events(event registration refnum=w39, error in=w37) -> (error out=w40:errorcluster)
  n235 = Merge Errors(w40, w42, w27) -> (w41:errorcluster)
  n236 = call "Destroy User Event - Stop.vi"("error in (no error)"=w41, "User Event - Stop"=w35) -> ("error out"=w30:errorcluster)  [unwired: 9 in]
  n237 = Release Notifier(notifier=w28, error in (no error)=w30) -> (error out=w29:errorcluster)  [unwired: 1 in, 2 out]
  n238 = disable-structure shown="RUN_TIME_ENGINE==True" {
    disable-tunnel: w29 -> [_ _]
    frame condition #0 (active) {
    }
    frame condition #1 {
      n239 = local read "Shutdown?"() -> (w528:bool)
      n240 = case shown="True" w528 {
        tunnel: [_ w530] -> w529
        frame False {
        }
        frame True {
          n241 = call <vilib>:"System Exec.vi"("wait until completion? (T)"=TRUE, "command line"="Shutdown -s -f -t 10") -> ("error out"=w530:errorcluster)  [unwired: 6 in, 3 out]
        }
      }
      n242 = flat-sequence {
        tunnel: w529 -> [_]
        frame #0 {
          n243 = Quit LabVIEW() -> ()  [unwired: 1 in]
        }
      }
    }
  }
